vi "parse.issue.side_panel.vi"(8 "error in (no error)":errorcluster, 10 "body":string, 11 "issue_class in":refnum<class "issue_class.lvclass">) -> (0 "error out":errorcluster, 3 "issue_class out":refnum<class "issue_class.lvclass">)   [LabVIEW 2024, in "issue_class.lvclass"]
uses:
  issue_class.lvclass
  issue_class.lvclass/issue_class.ctl
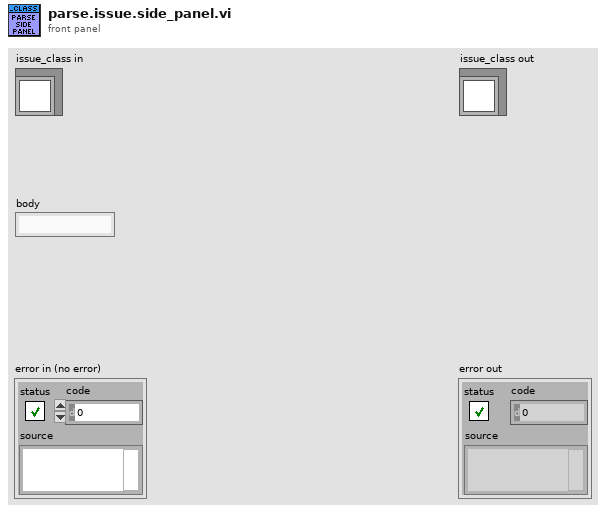
[diagram p1: front panel]
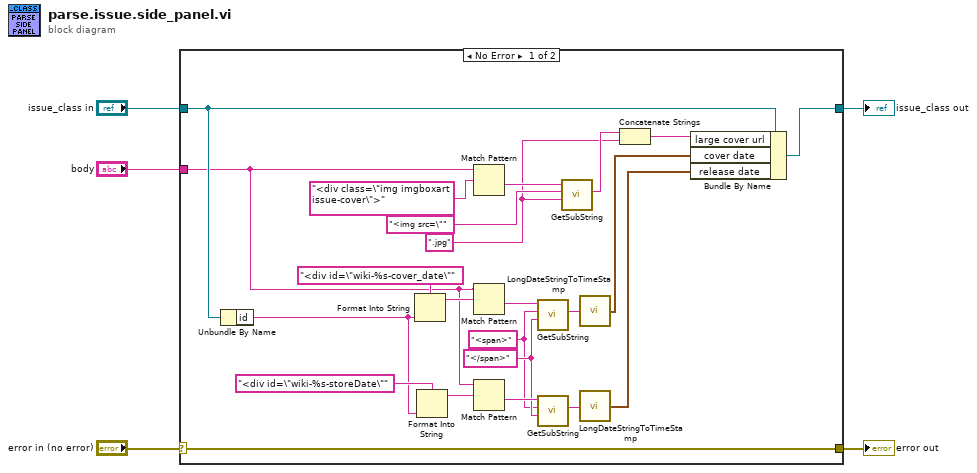
[diagram p0: block diagram]
diagram:
  n1 = case shown="No Error" "error in (no error)" {
    selector: "error in (no error)" -> [w28 w30]
    tunnel: [w28 w30] -> w4
    tunnel: [w24 w29] -> w2
    tunnel: "issue_class in" -> [w23 w29]
    tunnel: "body" -> [w15 _]
    frame No Error {
      w12 = "</span>" ("Start Search")
      w11 = "<span>" ("Start Search")
      w6 = ".jpg" ("End Search")
      n2 = Unbundle By Name(w23) -> ("id"=w20:string)
      n3 = Format Into String(format string="<div id=\"wiki-%s-cover_date\"" ("Start Search"), w20) -> (resulting string=w19:string)  [unwired: 2 in, 1 out]
      n4 = Format Into String(format string="<div id=\"wiki-%s-storeDate\"" ("Start Search"), w20) -> (resulting string=w14:string)  [unwired: 2 in, 1 out]
      n5 = Match Pattern(string=w15, regular expression="<div class=\"img imgboxart issue-cover\">") -> (after substring=w26:string)  [unwired: 1 in, 3 out]
      n6 = Match Pattern(string=w15, regular expression=w19) -> (after substring=w18:string)  [unwired: 1 in, 3 out]
      n7 = Match Pattern(string=w15, regular expression=w14) -> (after substring=w13:string)  [unwired: 1 in, 3 out]
      n8 = call "GetSubString.vi"("End Search"=w12, "Start Search"=w11, "String In"=w18) -> ("Match"=w17:string)  [unwired: 6 in, 2 out]
      n9 = call "GetSubString.vi"("End Search"=w12, "Start Search"=w11, "String In"=w13) -> ("Match"=w10:string)  [unwired: 6 in, 2 out]
      n10 = call "GetSubString.vi"("End Search"=w6, "Start Search"="<img src=\"", "String In"=w26) -> ("Match"=w7:string)  [unwired: 6 in, 2 out]
      n11 = call "LongDateStringToTimeStamp.vi"("long date string"=w17) -> ("time stamp"=w16:timestamp)
      n12 = call "LongDateStringToTimeStamp.vi"("long date string"=w10) -> ("time stamp"=w9:timestamp)
      n13 = Concatenate Strings(w7, w6) -> (w8:string)
      n14 = Bundle By Name(cluster=w23, "large cover url"=w8, "cover date"=w16, "release date"=w9) -> (w24:refnum<class "issue_class.lvclass">)
    }
    frame Error {
    }
  }
  "error out" <- w4
  "issue_class out" <- w2
